vi "ziSweeperPtByPt.vi"(0 "Handle In":T2 {"Handle" format="0x%08x"; "Conn" format="0x%08x"}, 1 "Output Demod (0)":u16, 2 "Signal Output (0)":u16 max=1, 3 "Averaging":u16(ring)=1 caption="Averaging (1)" items=["1"=1, "2"=2, "4"=4, "8"=8, "16"=16, "32"=32, "64"=64, "128"=128], 5 "Sweep Sequence In":dbl[][](array[numeric]) format="%#_6p", 7 "State In":T1 {"Output (F,X1,Y1,X2,Y2,...,Vo)" format="%#_4p"}, 9 "Oscillator (0)":u16, 11 "Error In":errorcluster, 12 "Input Demods (0)":u16[](array[numeric])=[0], 13 "Harmonic (1=fundamental)":i32=1 min=1 max=66000, 14 "Order (4)":i32(ring)=4 items=["6, 1st"=1, "12, 2nd"=2, "18, 3rd"=3, "24, 4th"=4, "30, 5th"=5, "36, 6th"=6, "42, 7th"=7, "48, 8th"=8]) -> (4 "Handle Out":T2 {"Handle" format="0x%08x"; "Conn" format="0x%08x"}, 8 "State Out":T1 {"Output (F,X1,Y1,X2,Y2,...,Vo)" format="%#_4p"}, 10 "Done":bool, 15 "Error Out":errorcluster)   [LabVIEW 2016, in "Zurich Instruments LabOne.lvlib"]
doc: "Perform a frequency sweep with the speciefied paramters. Use <B>ziSweepGenerator.vi</B> to generate the <B>Sweep Sequence</B>.\n\n<B>Output Channel</B> selects the channel in the output mixer that is used to generate the signal. This also determines the respective demodulator for generation of a sinusoidal.\n\nNote: <B>Signal Input</B> is only supported with the HF2LI when the Multifrequency option is installed."
uses:
  Zurich Instruments LabOne.lvlib
  ziTypeHandle.ctl
  ziTicksToS_single.vi
panel:
  out "Graph":cluster{dbl[], dbl[]}[](graph)
  in  "Abort":bool
  out "Remaining settle (s)":dbl caption="time to next value"
  out "Frequency":dbl caption="Frequency (Hz)" format="%_7p"
  out "Progress":dbl(slide) scale=0.0..1.0
  out "Bandwidth_indic":dbl=100.0 caption="Bandwidth (Hz)" format="%_3p"
  # "Status"
  # "Progress (%)"
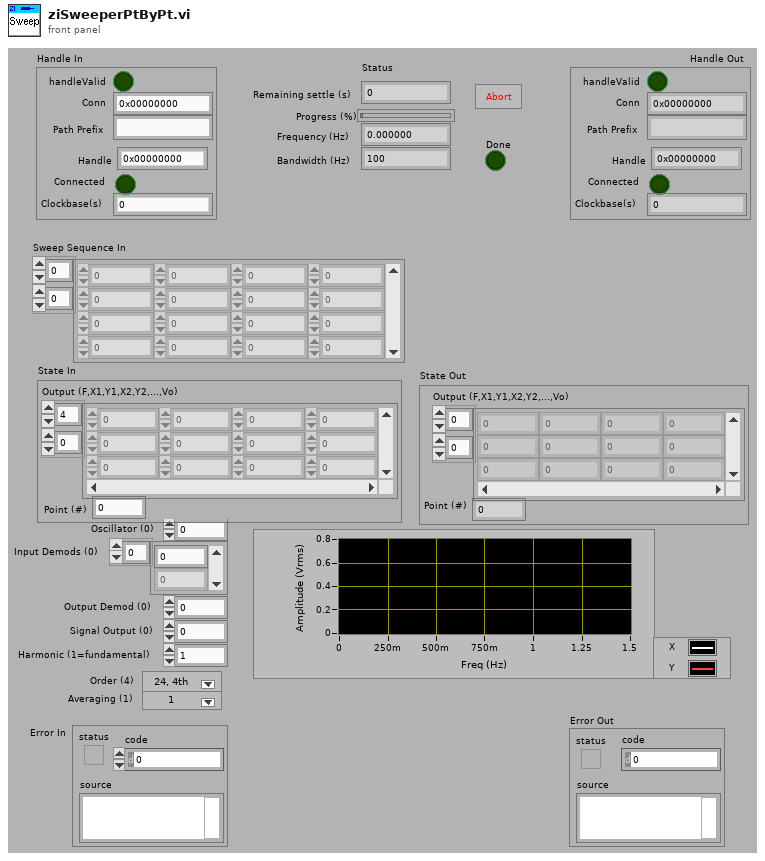
[diagram p1: front panel]
types:
  T1 = cluster{"Output (F,X1,Y1,X2,Y2,...,Vo)":dbl[][], "Point (#)":i32}
  T2 = typedef "Zurich Instruments LabOne.lvlib/ziTypeHandle.ctl" = cluster{"handleValid":bool, "Conn":u64, "Path Prefix":string, "Handle":u64, "Connected":bool, "Clockbase(s)":dbl}
  T3 = cluster{"Timestamps (ticks)":u64, "X (Vrms)":dbl, "Y (Vrms)":dbl, "Osc Phase (deg)":dbl, "Freq (Hz)":dbl, "DIO":u32, "AuxIn0 (V)":dbl, "AuxIn1 (V)":dbl}
  T4 = cluster{"Output (F,X1,Y1,X2,Y2,...,Vo)":dbl[], "Output (F,X1,Y1,X2,Y2,...,Vo)":dbl[]}
  T5 = cluster{"Output (F,X1,Y1,X2,Y2,...,Vo)":dbl[], "Output (F,X1,Y1,X2,Y2,...,Vo)":dbl[]}[]
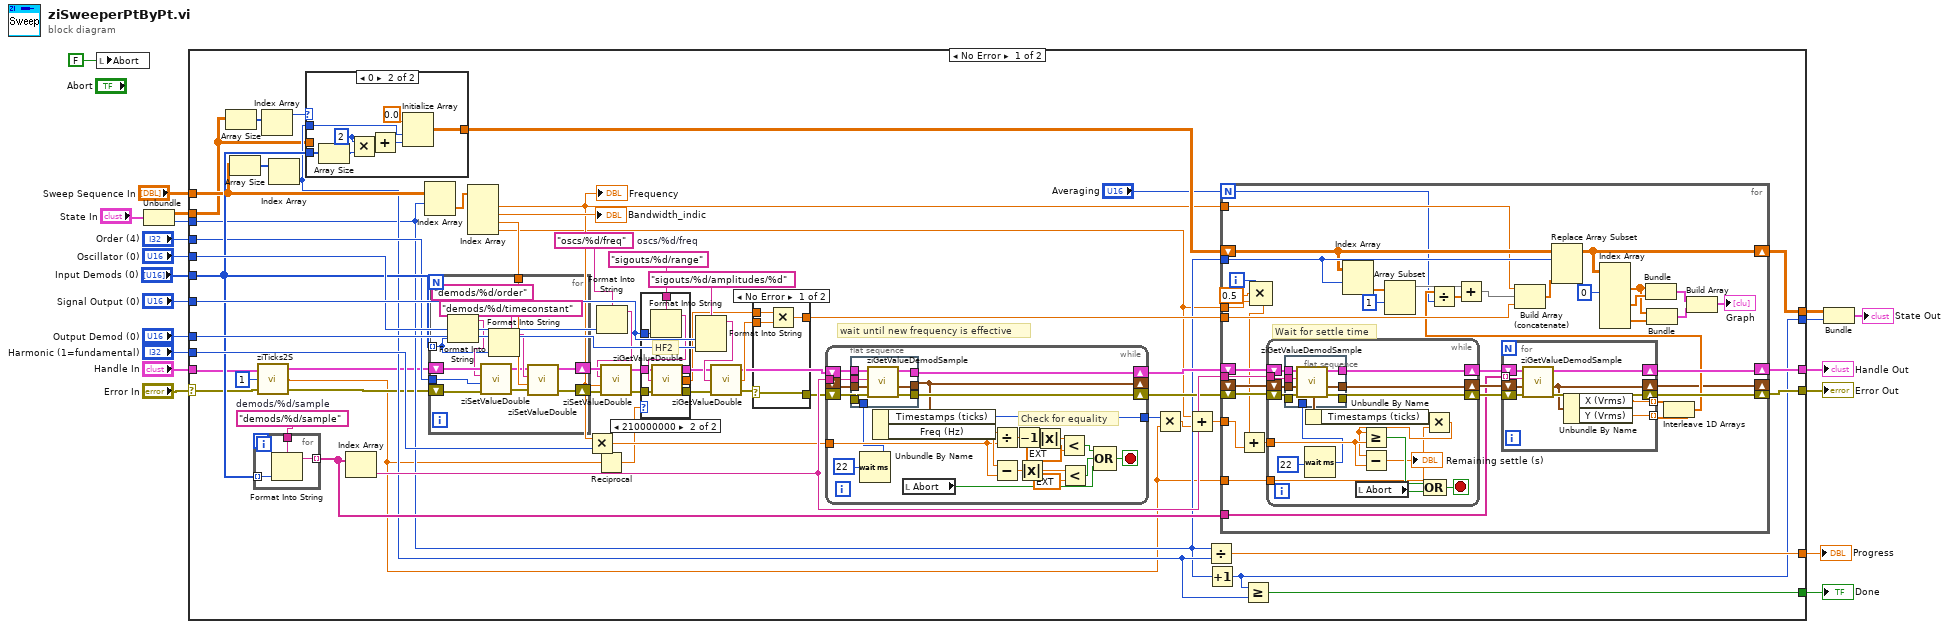
[diagram p0: block diagram]
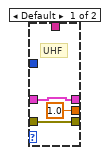
[diagram p2: hidden frame]
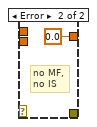
[diagram p3: hidden frame]
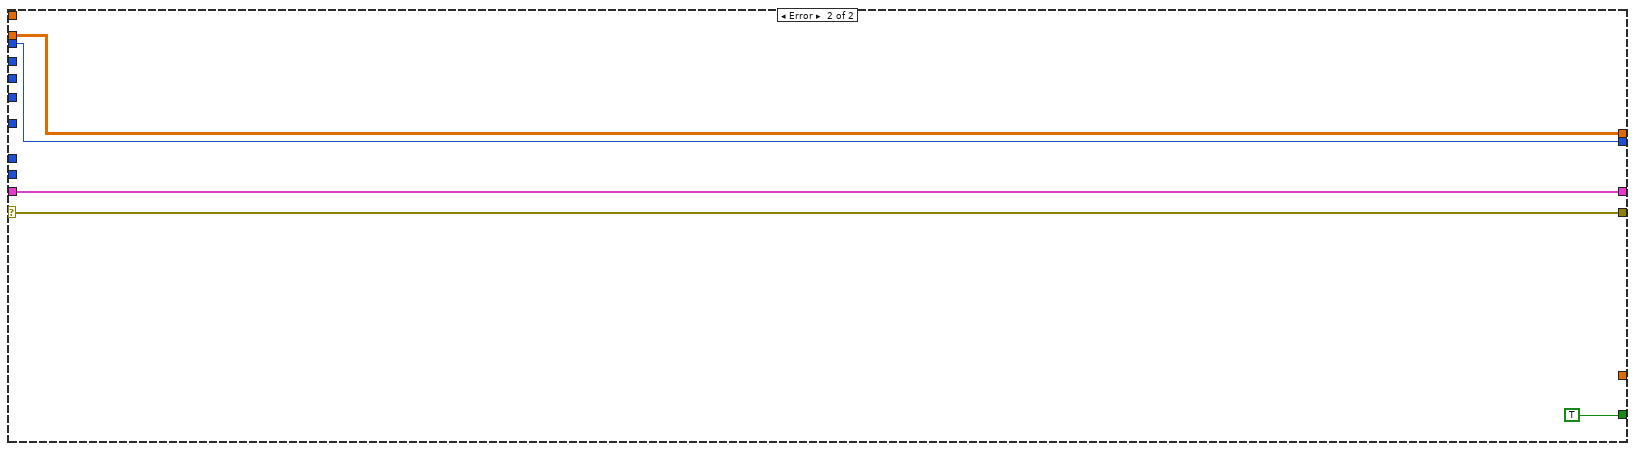
[diagram p5: hidden frame]
diagram:
  n1 = local write "Abort"(FALSE ("Abort")) -> ()
  n2 = Unbundle("State In") -> ("Output (F,X1,Y1,X2,Y2,...,Vo)"=w3:dbl[][], "Point (#)"=w2:i32)
  n3 = case shown="No Error" "Error In" {
    selector: "Error In" -> [w28 w227]
    tunnel: "Signal Output (0)" -> [w77 _]
    tunnel: "Output Demod (0)" -> [w76 _]
    tunnel: [w75 w228] -> w17
    tunnel: [w74 w227] -> w16
    tunnel: "Oscillator (0)" -> [w73 _]
    tunnel: "Harmonic (1=fundamental)" -> [w72 _]
    tunnel: "Input Demods (0)" -> [w66 _]
    tunnel: [w61 _] -> w12
    tunnel: "Handle In" -> [w29 w228]
    tunnel: [w44 TRUE] -> w10
    tunnel: "Order (4)" -> [w43 _]
    tunnel: "Sweep Sequence In" -> [w40 _]
    tunnel: [w37 w225] -> w7
    tunnel: [w36 w224] -> w6
    tunnel: w3 -> [w35 w225]
    tunnel: w2 -> [w34 w224]
    frame No Error {
      w55 = "oscs/%d/freq"  # oscs/%d/freq
      w69 = "demods/%d/sample"  # demods/%d/sample
      # "wait until new frequency is effective"
      n4 = Array Size(array=w35) -> (size(s)=w42:i32[])
      n5 = Array Size(array=w40) -> (size(s)=w39:i32[])
      n6 = for {
        tunnel: w69 -> [w223]
        tunnel: w66 -> [w222] mode=indexing
        tunnel: [w221] -> w67 mode=indexing
        n7 = Format Into String(format string=w223, w222) -> (resulting string=w221:string)  [unwired: 2 in, 1 out]
      }
      n8 = call-poly "ziTicks2S.vi"("Error In"=w28, "Timestamp(ticks)"=u64 1, "Handle In"=w29) -> ("Error Out"=w27:errorcluster, "Timestamp(s)"=w25:dbl, "Handle Out"=w26:T2)
      n9 = Index Array(array=w42) -> (element=w41:i32)  [unwired: 1 in]
      n10 = Index Array(array=w39) -> (element=w38:i32)  [unwired: 1 in]
      n11 = case shown="0" w41 {
        tunnel: [w96 w103] -> w79
        tunnel: w66 -> [_ w101]
        tunnel: w35 -> [w96 _]
        tunnel: w38 -> [_ w97]
        frame Default {
        }
        frame 0 {
          w98 = 2 ("dimension size")
          n12 = Array Size(array=w101) -> (size(s)=w100:i32)
          n13 = Multiply(x=w98, y=w100) -> (x*y=w99:i32)
          n14 = Add(x=w98, y=w99) -> (x+y=w102:i32)
          n15 = Initialize Array(0.0 ("dimension size"), w97, w102) -> (w103:dbl[][])
        }
      }
      n16 = Index Array(array=w67) -> (element=w68:string)  [unwired: 1 in]
      n17 = Index Array(array=w40, index (row)=w34) -> (element=w45:dbl[])  [unwired: 1 in]
      n18 = Index Array(array=w45) -> (element #1=w59:dbl, element #2=→"Bandwidth_indic":dbl, element #3=w58:dbl, element #4=w21:dbl)  [unwired: 4 in]
      "Frequency" <- w59
      n19 = for {
        tunnel: w66 -> [w105] mode=indexing
        tunnel: w58 -> [w117]
        shift-right: [w114] -> w53
        shift-left: w26 -> [w110]
        shift-right: [w113] -> w52
        shift-left: w27 -> [w111]
        tunnel: w43 -> [w108]
        n20 = Format Into String(format string="demods/%d/order", w105) -> (resulting string=w106:string)  [unwired: 2 in, 1 out]
        n21 = call "ziSetValueDouble.vi"("Error In"=w111, "Value"=w108, "Path"=w106, "Handle In"=w110) -> ("Error Out"=w112:errorcluster, "Handle Out"=w109:T2)  [unwired: 1 in]
        n22 = Format Into String(format string="demods/%d/timeconstant", w105) -> (resulting string=w115:string)  [unwired: 2 in, 1 out]
        n23 = call "ziSetValueDouble.vi"("Error In"=w112, "Value"=w117, "Path"=w115, "Handle In"=w109) -> ("Error Out"=w113:errorcluster, "Handle Out"=w114:T2)  [unwired: 1 in]
      }
      n24 = Multiply(x=w59, y=w72) -> (x*y=w54:dbl)
      n25 = Reciprocal(x=w25) -> (1/x=w24:dbl)
      n26 = Format Into String(format string=w55, w73) -> (resulting string=w51:string)  [unwired: 2 in, 1 out]
      n27 = call "ziSetValueDouble.vi"("Error In"=w52, "Value"=w59, "Path"=w51, "Handle In"=w53) -> ("Error Out"=w46:errorcluster, "Handle Out"=w47:T2)  [unwired: 1 in]
      n28 = case shown="210000000" w24 {
        tunnel: "sigouts/%d/range" -> [_ w89]
        tunnel: w77 -> [_ w88]
        tunnel: [w80 w87] -> w65
        tunnel: [w82 w86] -> w64
        tunnel: [1.0 ("Value") w85] -> w62
        tunnel: w47 -> [w80 w84]
        tunnel: w46 -> [w82 w83]
        frame Default {
          # "UHF"
        }
        frame 210000000 {
          # "HF2"
          n29 = Format Into String(format string=w89, w88) -> (resulting string=w90:string)  [unwired: 2 in, 1 out]
          n30 = call "ziGetValueDouble.vi"("error in"=w83, "Path"=w90, "Handle in"=w84) -> ("error out"=w86:errorcluster, "Value"=w85:dbl, "Handle out"=w87:T2)
        }
      }
      n31 = Format Into String(format string="sigouts/%d/amplitudes/%d", w77, w76) -> (resulting string=w71:string)  [unwired: 2 in, 1 out]
      n32 = call "ziGetValueDouble.vi"("error in"=w64, "Path"=w71, "Handle in"=w65) -> ("error out"=w33:errorcluster, "Value"=w63:dbl, "Handle out"=w48:T2)
      n33 = case shown="No Error" w33 {
        selector: w33 -> [w91 _]
        tunnel: w63 -> [w94 _]
        tunnel: w62 -> [w93 _]
        tunnel: [w92 0.0] -> w49
        tunnel: [w91 _] -> w32
        frame No Error {
          n34 = Multiply(x=w93, y=w94) -> (x*y=w92:dbl)
        }
        frame Error {
          # "no MF,\nno IS"
        }
      }
      n35 = while {
        tunnel: w54 -> [w197]
        tunnel: [w191] -> w31
        shift-right: [w209] -> w56
        shift-left: w48 -> [w212]
        shift-right: [w208] -> w57
        shift-left: w32 -> [w211]
        tunnel: w68 -> [w207]
        shift-right: [w201] -> _
        shift-left: _ -> [w200]
        stop <- w213 stop-if-true
        # "Check for equality"
        n36 = flat-sequence {
          tunnel: w212 -> [w220]
          tunnel: w211 -> [w219]
          tunnel: [w218] -> w209
          tunnel: [w217] -> w208
          tunnel: w207 -> [w216]
          tunnel: [w215] -> w201
          tunnel: w200 -> [w214]
          tunnel: w192 -> [_]
          frame #0 {
            n37 = call "ziGetValueDemodSample.vi"("error in"=w219, "Demod Sample In"=w214, "Path"=w216, "Handle In"=w220) -> ("error out"=w217:errorcluster, "Demod Sample Out"=w215:T3, "Handle Out"=w218:T2)  [unwired: 1 in]
          }
        }
        n38 = Wait (ms)(milliseconds to wait=22 ("timeout in ms (-1)")) -> (millisecond timer value=w192:u32)
        n39 = Unbundle By Name(w201) -> ("Timestamps (ticks)"=w191:u64, "Freq (Hz)"=w198:dbl)
        n40 = local read "Abort"() -> (w206:bool)
        n41 = Divide(x=w198, y=w197) -> (x/y=w202:dbl)
        n42 = Subtract(x=w198, y=w197) -> (x-y=w196:dbl)
        n43 = Decrement(x=w202) -> (x-1=w203:dbl)
        n44 = Absolute Value(x=w196) -> (abs(x)=w194:dbl)
        n45 = Absolute Value(x=w203) -> (abs(x)=w204:dbl)
        n46 = Less?(x=w204, y=ext 1e-7) -> (x < y?=w199:bool)
        n47 = Less?(x=w194, y=ext 0.00001) -> (x < y?=w193:bool)
        n48 = Compound Arithmetic op=OR(w199, w193, w206) -> (w213:bool)
      }
      n49 = Multiply(x=w31, y=w25) -> (x*y=w23:dbl)
      n50 = Add(x=w21, y=w23) -> (x+y=w22:dbl)
      n51 = Divide(x=w34, y=w38) -> (x/y=w61:dbl)
      n52 = Increment(x=w34) -> (x+1=w36:i32)
      n53 = for {
        N: "Averaging" -> [w125]
        shift-right: [w135] -> w75
        shift-left: w56 -> [w157]
        shift-right: [w134] -> w74
        shift-left: w57 -> [w156]
        tunnel: w49 -> [w139]
        tunnel: w59 -> [w140]
        tunnel: w34 -> [w154]
        shift-right: [w148] -> w37
        shift-left: w79 -> [w153]
        tunnel: w68 -> [w149]
        tunnel: w67 -> [w133]
        shift-right: [w129] -> _
        shift-left: _ -> [w128]
        tunnel: w25 -> [w124]
        tunnel: w22 -> [w121]
        tunnel: w21 -> [w120]
        i -> [w123]
        # "Wait for settle time"
        n54 = Compound Arithmetic op=MULTIPLY(w123, 0.5 ("dimension size"), w120) -> (w119:dbl)
        n55 = Add(x=w119, y=w121) -> (x+y=w118:dbl)
        n56 = while {
          tunnel: w118 -> [w183]
          shift-right: [w180] -> w137
          shift-left: w156 -> [w181]
          shift-right: [w176] -> w138
          shift-left: w157 -> [w182]
          shift-right: [w174] -> w136
          shift-left: w128 -> [w175]
          tunnel: w149 -> [w172]
          tunnel: w124 -> [w167]
          stop <- w178 stop-if-true
          n57 = flat-sequence {
            tunnel: w182 -> [w190]
            tunnel: w181 -> [w189]
            tunnel: [w188] -> w180
            tunnel: [w187] -> w176
            tunnel: w175 -> [w186]
            tunnel: [w185] -> w174
            tunnel: w172 -> [w184]
            tunnel: w170 -> [_]
            frame #0 {
              n58 = call "ziGetValueDemodSample.vi"("error in"=w189, "Demod Sample In"=w186, "Path"=w184, "Handle In"=w190) -> ("error out"=w188:errorcluster, "Demod Sample Out"=w185:T3, "Handle Out"=w187:T2)  [unwired: 1 in]
            }
          }
          n59 = Wait (ms)(milliseconds to wait=22 ("timeout in ms (-1)")) -> (millisecond timer value=w170:u32)
          n60 = Unbundle By Name(w174) -> ("Timestamps (ticks)"=w168:u64)
          n61 = local read "Abort"() -> (w173:bool)
          n62 = Multiply(x=w168, y=w167) -> (x*y=w169:dbl)
          n63 = Greater Or Equal?(x=w169, y=w183) -> (x >= y?=w179:bool)
          n64 = Subtract(x=w169, y=w183) -> (x-y=→"Remaining settle (s)":dbl)
          n65 = Compound Arithmetic op=OR(w179, w173) -> (w178:bool)
        }
        n66 = Index Array(array=w153, index (row)=w154) -> (element=w152:dbl[])  [unwired: 1 in]
        n67 = Array Subset(array=w152, index=1) -> (w150:dbl[])  [unwired: 1 in]
        n68 = for {
          shift-right: [w163] -> w134
          shift-left: w137 -> [w164]
          shift-right: [w162] -> w135
          shift-left: w138 -> [w165]
          tunnel: [w166] -> w132 mode=indexing
          tunnel: [w159] -> w131 mode=indexing
          shift-right: [w160] -> w129
          shift-left: w136 -> [w161]
          tunnel: w133 -> [w158] mode=indexing
          n69 = call "ziGetValueDemodSample.vi"("error in"=w164, "Demod Sample In"=w161, "Path"=w158, "Handle In"=w165) -> ("error out"=w163:errorcluster, "Demod Sample Out"=w160:T3, "Handle Out"=w162:T2)  [unwired: 1 in]
          n70 = Unbundle By Name(w160) -> ("X (Vrms)"=w166:dbl, "Y (Vrms)"=w159:dbl)
        }
        n71 = Interleave 1D Arrays(w132, w131) -> (w130:dbl[])
        n72 = Divide(x=w130, y=w125) -> (x/y=w126:dbl[])
        n73 = Add(x=w150, y=w126) -> (x+y=w127:dbl[])
        n74 = Build Array (concatenate)(w140, w127, w139) -> (w155:dbl[])
        n75 = Replace Array Subset(array=w153, new element=w155, index (row)=w154) -> (w148:dbl[][])  [unwired: 1 in]
        n76 = Index Array(array=w148, index (col) #1=0 ("index (row)")) -> (element #1=w143:dbl[], element #2=w147:dbl[], element #3=w145:dbl[])  [unwired: 5 in]
        n77 = Bundle("Output (F,X1,Y1,X2,Y2,...,Vo)"=w143, "Output (F,X1,Y1,X2,Y2,...,Vo)"=w147) -> (w146:T4)  [unwired: 1 out]
        n78 = Bundle("Output (F,X1,Y1,X2,Y2,...,Vo)"=w143, "Output (F,X1,Y1,X2,Y2,...,Vo)"=w145) -> (w144:T4)  [unwired: 1 out]
        n79 = Build Array(w146, w144) -> (→"Graph":T5)
      }
      n80 = Greater Or Equal?(x=w36, y=w38) -> (x >= y?=w44:bool)
    }
    frame Error {
    }
  }
  "Handle Out" <- w17
  "Error Out" <- w16
  "Done" <- w10
  "Progress" <- w12
  n81 = Bundle("Output (F,X1,Y1,X2,Y2,...,Vo)"=w7, "Point (#)"=w6) -> (→"State Out":T1)  [unwired: 1 in]
